vi "GetBit(U64).vi"() -> ()   [LabVIEW 2011]
panel:
  out "Bit":bool
  out "Bit(0or1)":i16
  in  "Bit(0-63)":u8
  in  "Input(U8)":u64 format="%.0x"
  out "error out":errorcluster caption="错误输出"
  in  "error in (no error)":errorcluster caption="错误输入（无错误）"
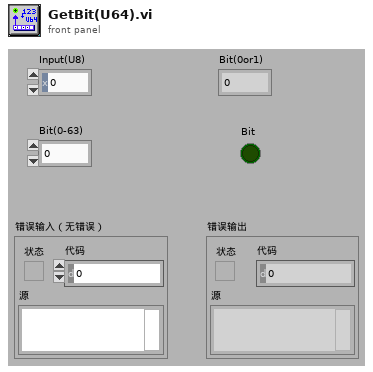
[diagram p1: front panel]
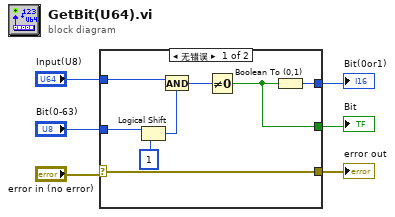
[diagram p0: block diagram]
diagram:
  n1 = case shown="无错误" "error in (no error)" {
    selector: "error in (no error)" -> [w14 w15]
    tunnel: [w14 w15] -> w5
    tunnel: "Bit(0-63)" -> [w13 _]
    tunnel: "Input(U8)" -> [w12 _]
    tunnel: [w10 _] -> w2
    tunnel: [w9 _] -> w1
    frame No Error {
      n2 = Logical Shift(y=w13, x=u64 1) -> (x << y=w7:u64)
      n3 = And(x=w12, y=w7) -> (x .and. y?=w11:u64)
      n4 = Not Equal To 0?(x=w11) -> (x != 0?=w10:bool)
      n5 = Boolean To (0,1)(Boolean=w10) -> (0, 1=w9:i16)
    }
    frame Error {
    }
  }
  "error out" <- w5
  "Bit" <- w2
  "Bit(0or1)" <- w1
